vi "Read Element of Axis-parameters.vi"(8 "error in (no error)":errorcluster, 10 "index":i32, 11 "DelayLine in":refnum<class "DelayLine.lvclass">) -> (0 "error out":errorcluster, 2 "Axis-Pos":T1, 3 "DelayLine out":refnum<class "DelayLine.lvclass">)   [LabVIEW 2016]
uses:
  DelayLine.lvclass
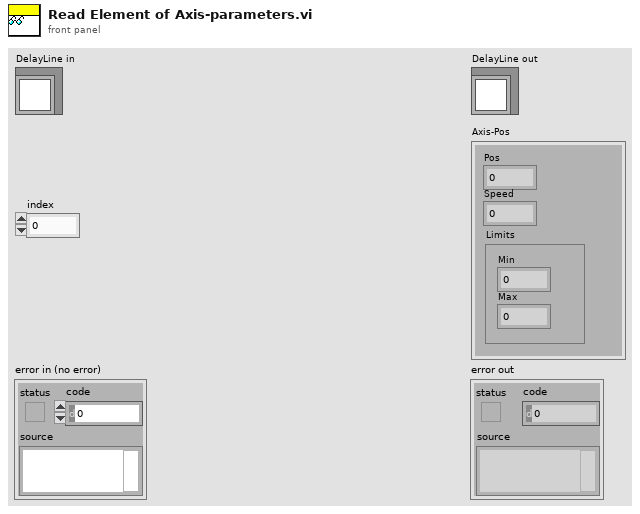
[diagram p1: front panel]
types:
  T1 = cluster{"Pos":dbl, "Speed":dbl, "Limits":cluster{"Min":dbl, "Max":dbl}}
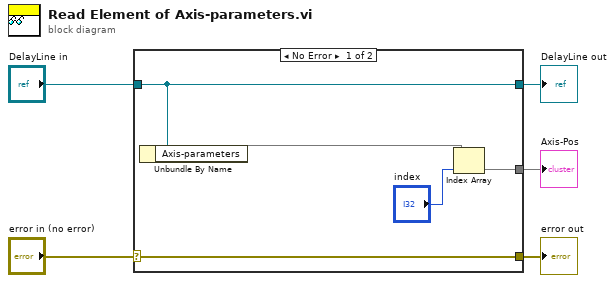
[diagram p0: block diagram]
diagram:
  n1 = case shown="No Error" "error in (no error)" {
    selector: "error in (no error)" -> [w10 w11]
    tunnel: [w10 w11] -> w4
    tunnel: [w9 w12] -> w2
    tunnel: "DelayLine in" -> [w9 w12]
    tunnel: [w6 _] -> w1
    frame No Error {
      n2 = Unbundle By Name(w9) -> ("Axis-parameters"=w8)
      n3 = Index Array(array=w8, index="index") -> (element=w6)
    }
    frame Error {
    }
  }
  "error out" <- w4
  "DelayLine out" <- w2
  "Axis-Pos" <- w1
